vi "cameraSwitchModeAndSetParams.vi"(2 "error in (no error)":errorcluster {"code" format="%.0x"}, 3 "Camera Handle":u32, 4 "Calculate\nExposure\nTimes":bool=TRUE) -> (0 "error out":errorcluster, 1 "Camera Handle Out":u32)   [LabVIEW 2013]
uses:
  cameraGlobal.vi
  ScanningParametersGlobal.vi
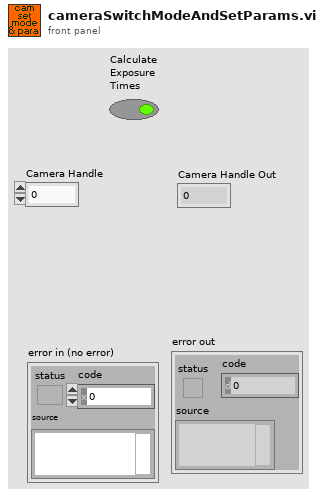
[diagram p1: front panel]
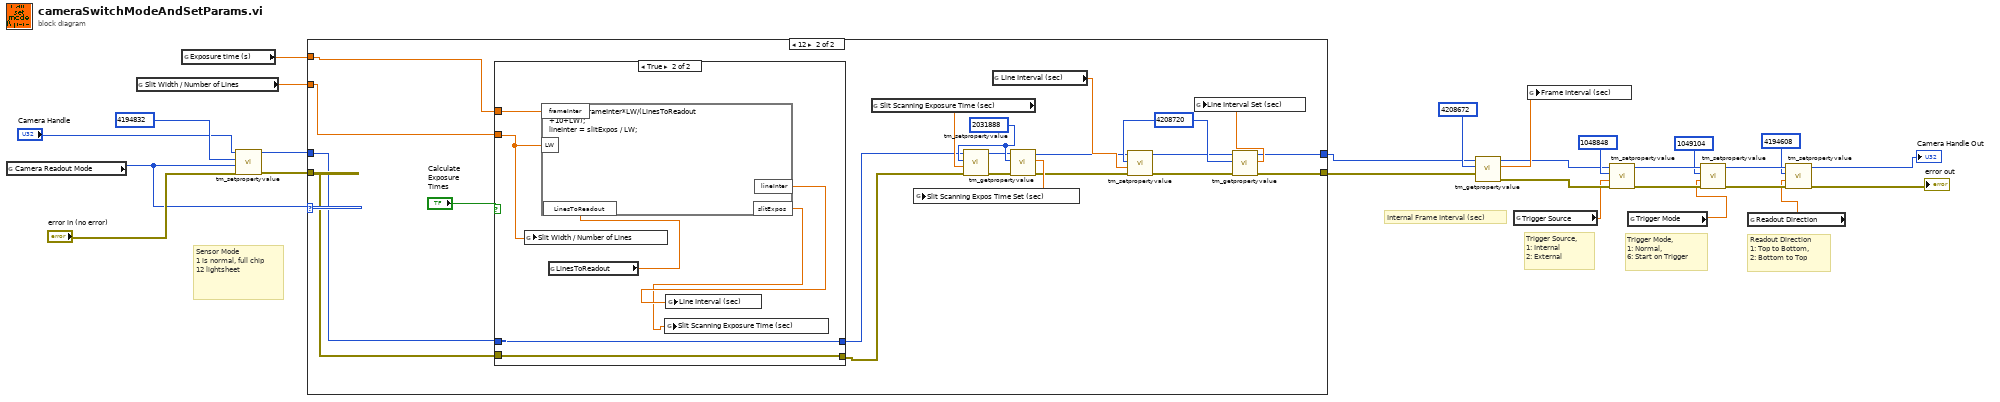
[diagram p0: block diagram]
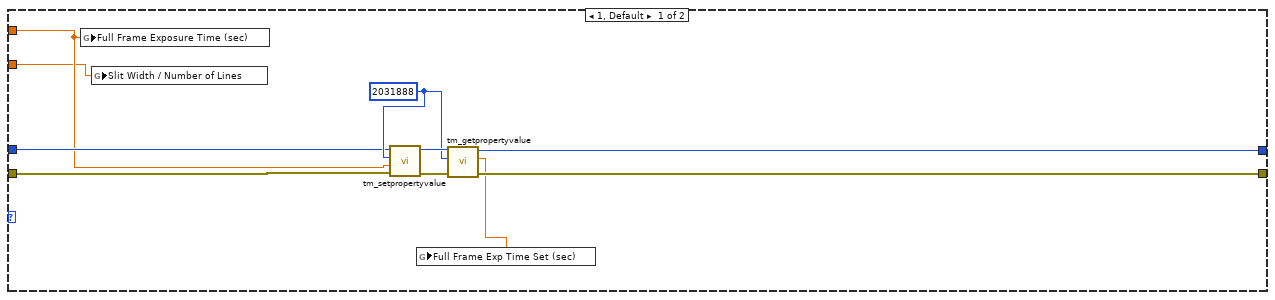
[diagram p2: hidden frame]
diagram:
  # "Internal Frame Interval (sec)"
  # "Sensor Mode \n1 is normal, full chip\n12 lightsheet"
  # "Readout Direction \n1: Top to Bottom, \n2: Bottom to Top"
  # "Trigger Mode, \n1: Normal, \n6: Start on Trigger"
  # "Trigger Source, \n1: Internal \n2: External"
  n1 = global read "cameraGlobal.vi" "Camera Readout Mode"() -> (w15:u16)
  n2 = global read "ScanningParametersGlobal.vi" "Slit Width / Number of Lines"() -> (w1:sgl)
  n3 = global read "ScanningParametersGlobal.vi" "Exposure time (s)"() -> (w2:dbl)
  n4 = call <userlib>:"tm_setpropertyvalue.vi"("error in (no error)"="error in (no error)", "Value in"=w15, "Property ID"=u32 4194832, "Handle in"="Camera Handle") -> ("error out"=w17:errorcluster, "Handle out"=w16:u32)  [unwired: 6 in]
  n5 = case shown="12" w15 {
    tunnel: w16 -> [w30 w42]
    tunnel: w17 -> [w29 w43]
    tunnel: [w35 w45] -> w12
    tunnel: [w36 w44] -> w11
    tunnel: w2 -> [w28 w38]
    tunnel: w1 -> [w27 w37]
    frame 1, Default {
      w32 = u32 2031888 ("Property ID")
      n6 = global write "cameraGlobal.vi" "Full Frame Exposure Time (sec)"(w28) -> ()
      n7 = global write "cameraGlobal.vi" "Slit Width / Number of Lines"(w27) -> ()
      n8 = call <userlib>:"tm_setpropertyvalue.vi"("error in (no error)"=w29, "Value in"=w28, "Property ID"=w32, "Handle in"=w30) -> ("error out"=w34:errorcluster, "Handle out"=w33:u32)  [unwired: 6 in]
      n9 = call <userlib>:"tm_getpropertyvalue.vi"("error in (no error)"=w34, "Property ID"=w32, "Handle in"=w33) -> ("error out"=w36:errorcluster, "Value in"=w31:sgl, "Handle out"=w35:u32)  [unwired: 6 in]
      n10 = global write "cameraGlobal.vi" "Full Frame Exp Time Set (sec)"(w31) -> ()
    }
    frame 12 {
      w54 = u32 4208720 ("Property ID")
      w57 = u32 2031888 ("Property ID")
      n11 = case shown="True" "Calculate\nExposure\nTimes" {
        tunnel: w43 -> [w58 w63]
        tunnel: w42 -> [w59 w64]
        tunnel: [w59 w64] -> w41
        tunnel: [w58 w63] -> w40
        tunnel: w38 -> [_ w61]
        tunnel: w37 -> [_ w60]
        frame False {
        }
        frame True {
          n12 = global write "cameraGlobal.vi" "Slit Width / Number of Lines"(w60) -> ()
          n13 = global read "cameraGlobal.vi" "LinesToReadout"() -> (w62:sgl)
          n14 = formula code="slitExpos=frameInter*LW/(LinesToReadout\n+10+LW);\nlineInter = slitExpos / LW;"("frameInter"=w61, "LW"=w60, "LinesToReadout"=w62) -> ("slitExpos"=w65:dbl, "lineInter"=w66:dbl)
          n15 = global write "cameraGlobal.vi" "Slit Scanning Exposure Time (sec)"(w65) -> ()
          n16 = global write "cameraGlobal.vi" "Line Interval (sec)"(w66) -> ()
        }
      }
      n17 = global read "cameraGlobal.vi" "Slit Scanning Exposure Time (sec)"() -> (w51:dbl)
      n18 = call <userlib>:"tm_setpropertyvalue.vi"("error in (no error)"=w40, "Value in"=w51, "Property ID"=w57, "Handle in"=w41) -> ("error out"=w56:errorcluster, "Handle out"=w55:u32)  [unwired: 6 in]
      n19 = global read "cameraGlobal.vi" "Line Interval (sec)"() -> (w49:sgl)
      n20 = call <userlib>:"tm_getpropertyvalue.vi"("error in (no error)"=w56, "Property ID"=w57, "Handle in"=w55) -> ("error out"=w47:errorcluster, "Value in"=w50:sgl, "Handle out"=w48:u32)  [unwired: 6 in]
      n21 = global write "cameraGlobal.vi" "Slit Scanning Expos Time Set (sec)"(w50) -> ()
      n22 = call <userlib>:"tm_setpropertyvalue.vi"("error in (no error)"=w47, "Value in"=w49, "Property ID"=w54, "Handle in"=w48) -> ("error out"=w52:errorcluster, "Handle out"=w53:u32)  [unwired: 6 in]
      n23 = call <userlib>:"tm_getpropertyvalue.vi"("error in (no error)"=w52, "Property ID"=w54, "Handle in"=w53) -> ("error out"=w44:errorcluster, "Value in"=w46:sgl, "Handle out"=w45:u32)  [unwired: 6 in]
      n24 = global write "cameraGlobal.vi" "Line Interval Set (sec)"(w46) -> ()
    }
  }
  n25 = call <userlib>:"tm_getpropertyvalue.vi"("error in (no error)"=w11, "Property ID"=u32 4208672, "Handle in"=w12) -> ("error out"=w9:errorcluster, "Value in"=w13:sgl, "Handle out"=w10:u32)  [unwired: 6 in]
  n26 = global read "cameraGlobal.vi" "Trigger Source"() -> (w8:sgl)
  n27 = global write "cameraGlobal.vi" "Frame Interval (sec)"(w13) -> ()
  n28 = call <userlib>:"tm_setpropertyvalue.vi"("error in (no error)"=w9, "Value in"=w8, "Property ID"=u32 1048848, "Handle in"=w10) -> ("error out"=w22:errorcluster, "Handle out"=w26:u32)  [unwired: 6 in]
  n29 = global read "cameraGlobal.vi" "Trigger Mode"() -> (w7:sgl)
  n30 = call <userlib>:"tm_setpropertyvalue.vi"("error in (no error)"=w22, "Value in"=w7, "Property ID"=u32 1049104, "Handle in"=w26) -> ("error out"=w24:errorcluster, "Handle out"=w25:u32)  [unwired: 6 in]
  n31 = global read "cameraGlobal.vi" "Readout Direction"() -> (w6:sgl)
  n32 = call <userlib>:"tm_setpropertyvalue.vi"("error in (no error)"=w24, "Value in"=w6, "Property ID"=u32 4194608, "Handle in"=w25) -> ("error out"=→"error out":errorcluster, "Handle out"=→"Camera Handle Out":u32)  [unwired: 6 in]
